vi "phi_du.vi"(2 "error in (no error)":errorcluster, 3 "u_m":dbl, 4 "phi_d":T1) -> (0 "error out":errorcluster, 1 "phi_du":T1)   [LabVIEW 2021]
uses:
  <vilib>/Analysis/Matrix/Datatypes/RealMatrix.ctl
  <vilib>/Analysis/Matrix/NI_Matrix.lvlib
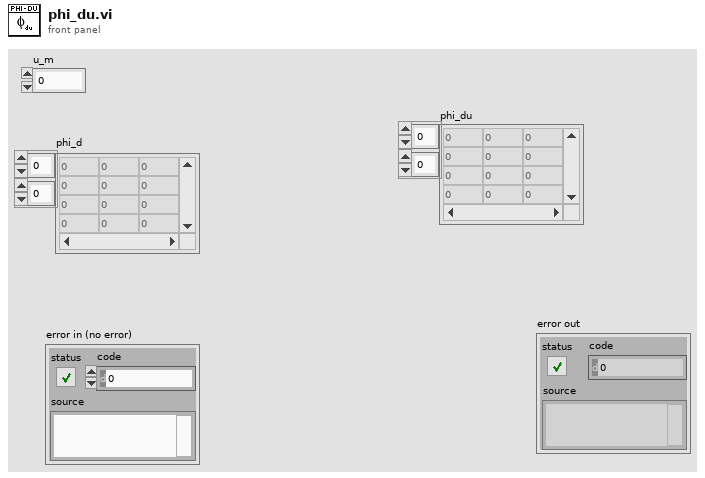
[diagram p1: front panel]
types:
  T1 = typedef "NI_Matrix.lvlib/RealMatrix.ctl" = dbl[][]
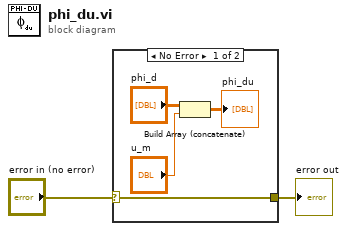
[diagram p0: block diagram]
diagram:
  n1 = case shown="No Error" "error in (no error)" {
    selector: "error in (no error)" -> [w3 w7]
    tunnel: [w3 w7] -> w1
    frame No Error {
      n2 = Build Array (concatenate)("phi_d", "u_m") -> (→"phi_du":T1)
    }
    frame Error {
    }
  }
  "error out" <- w1
